vi "PathPlanner_PathSegment_GetSegmentPoints.vi"(11 "Segment":T5 {"SegmentPoints"."HolonomicRotation"."SIN" format="%13.4f"; "SegmentPoints"."HolonomicRotation"."COS" format="%13.4f"; "SegmentPoints"."HolonomicRotation"."VALUE" format="%13.4f"; "SegmentPoints"."Position"."Y" format="%14.3f"; "SegmentPoints"."Position"."X" format="%14.3f"}) -> (3 "SegmentPoints":T1[](array[typedef]) {"HolonomicRotation"."SIN" format="%13.4f"; "HolonomicRotation"."COS" format="%13.4f"; "HolonomicRotation"."VALUE" format="%13.4f"; "Position"."Y" format="%14.3f"; "Position"."X" format="%14.3f"})   [LabVIEW 2019, in "PathPlanner.lvlib"]
doc: "Get the path points for this segment\n \nInputs: \n - PathSegment - cluster - Data defining path segment\n\nOutputs:\n - SetmentPoint - array - points for this segment"
uses:
  PathPlanner.lvlib
  TypeDef/PathPlannerPathSegment.ctl
  TypeDef/PathPlannerPathPoint.ctl
  <vilib>/Rock Robotics/WPI/ThirdParty/JAS_Junk/TrajLib/TypeDef/TRANSLATION2D.ctl
  <vilib>/Rock Robotics/WPI/ThirdParty/JAS_Junk/TrajLib/TypeDef/ROTATION2D.ctl
  TypeDef/PathPlannerPathConstraints.ctl
  <vilib>/Rock Robotics/WPI/ThirdParty/JAS_Junk/TrajLib/Trajectory_Library.lvlib
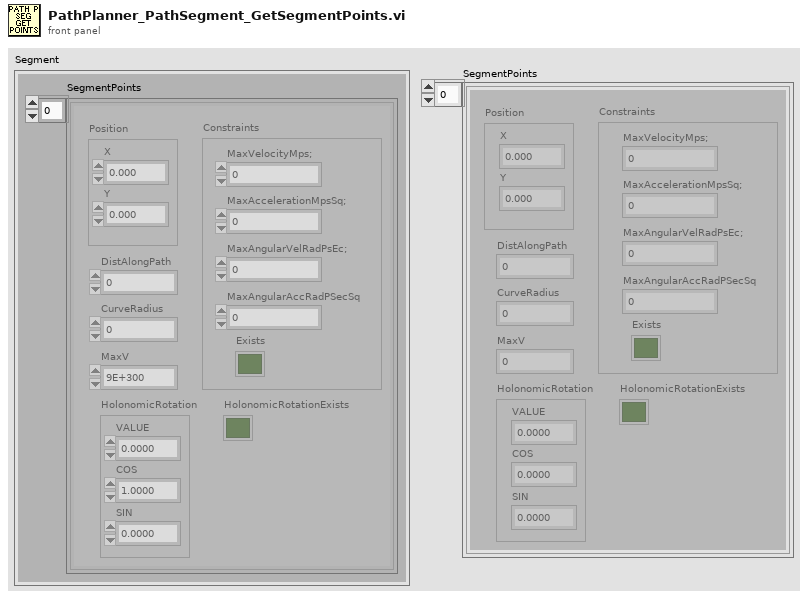
[diagram p1: front panel]
types:
  T1 = typedef "PathPlanner.lvlib/PathPlannerPathPoint.ctl" = cluster{"Position":T2, "HolonomicRotation":T3, "DistAlongPath":dbl, "CurveRadius":dbl, "MaxV":dbl, "Constraints":T4, "HolonomicRotationExists":bool}
  T2 = typedef "Trajectory_Library.lvlib/TRANSLATION2D.ctl" = cluster{"X":dbl, "Y":dbl}
  T3 = typedef "Trajectory_Library.lvlib/ROTATION2D.ctl" = cluster{"VALUE":dbl, "COS":dbl, "SIN":dbl}
  T4 = typedef "PathPlanner.lvlib/PathPlannerPathConstraints.ctl" = cluster{"MaxVelocityMps;":dbl, "MaxAccelerationMpsSq;":dbl, "MaxAngularVelRadPsEc;":dbl, "MaxAngularAccRadPSecSq":dbl, "Exists":bool}
  T5 = typedef "PathPlanner.lvlib/PathPlannerPathSegment.ctl" = cluster{"SegmentPoints":T1[]}
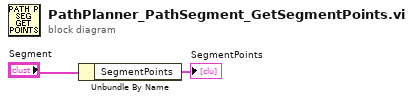
[diagram p0: block diagram]
diagram:
  n1 = Unbundle By Name("Segment") -> ("SegmentPoints"=→"SegmentPoints":T1[])
